vi "render hold note_pink.vi"(4 "head index":i32, 6 "progress":dbl, 7 "y-center":dbl, 10 "rail":cluster{"note type":string, "position":dbl}[](array[cluster]), 11 "new picture in":picture) -> (3 "new picture out":picture)   [LabVIEW 2023]
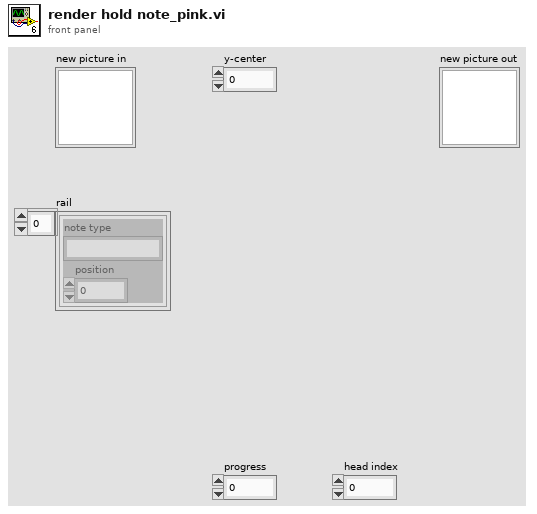
[diagram p1: front panel]
types:
  T1 = cluster{"Width":u16, "Style":enum32{"Solid", "Dash", "Dot", "DashDot", "DashDotDot"}}
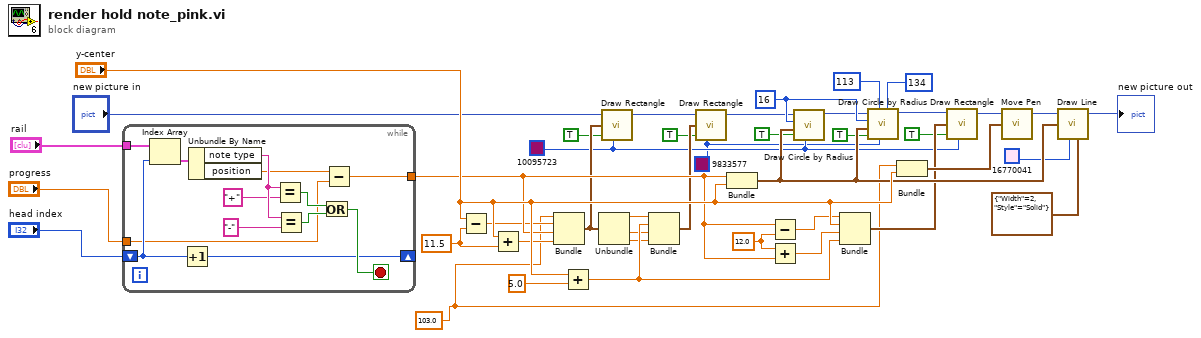
[diagram p0: block diagram]
diagram:
  w1 = 103.0 ("y")
  w4 = u32 9833577 ("color(black)")
  w5 = u32 10095723 ("color(black)")
  w31 = 12.0 ("y")
  w11 = 11.5 ("y")
  w28 = i16 16 ("radius")
  n1 = while {
    tunnel: "rail" -> [w55]
    shift-right: [w46] -> _
    shift-left: "head index" -> [w47]
    tunnel: "progress" -> [w45]
    tunnel: [w43] -> w32
    stop <- w48 stop-if-true
    n2 = Index Array(array=w55, index=w47) -> (element=w54:cluster{"note type":string, "position":dbl})
    n3 = Increment(x=w47) -> (x+1=w46:i32)
    n4 = Unbundle By Name(w54) -> ("note type"=w51:string, "position"=w44:dbl)
    n5 = Equal?(x=w51, y="+") -> (x = y?=w53:bool)
    n6 = Equal?(x=w51, y="-") -> (x = y?=w52:bool)
    n7 = Or(x=w53, y=w52) -> (x .or. y?=w48:bool)
    n8 = Subtract(x=w44, y=w45) -> (x-y=w43:dbl)
  }
  n9 = Subtract(x="y-center", y=w11) -> (x-y=w10:dbl)
  n10 = Add(x="y-center", y=w11) -> (x+y=w12:dbl)
  n11 = Bundle("y"=w1, w10, w32, w12) -> (w18:cluster{"y":dbl, dbl, dbl, dbl})  [unwired: 1 in]
  n12 = Add(x="y-center", y=5.0) -> (x+y=w35:dbl)
  n13 = Unbundle(w18) -> ("y"=w19:dbl, w20:dbl, w21:dbl)  [unwired: 1 out]
  n14 = call <vilib>:"Draw Rectangle.vi"("picture"="new picture in", "rect"=w18, "fill?(F)"=TRUE, "color(black)"=w5) -> ("new picture"=w15:picture)  [unwired: 5 in]
  n15 = Bundle("y"=w19, w35, w20, w21) -> (w23:cluster{"y":dbl, dbl, dbl, dbl})  [unwired: 1 in]
  n16 = call <vilib>:"Draw Rectangle.vi"("picture"=w15, "rect"=w23, "fill?(F)"=TRUE, "color(black)"=w4) -> ("new picture"=w16:picture)  [unwired: 5 in]
  n17 = Bundle(w32, "y-center"="y-center") -> (w40:cluster{dbl, "y-center":dbl})  [unwired: 1 in]
  n18 = Subtract(x=w32, y=w31) -> (x-y=w33:dbl)
  n19 = Add(x=w31, y=w32) -> (x+y=w34:dbl)
  n20 = call <vilib>:"Draw Circle by Radius.vi"("color(black)"=w5, "fill?(F)"=TRUE, "pixel center"=w40, "radius"=w28, "picture"=w16) -> ("new picture"=w24:picture)  [unwired: 6 in]
  n21 = Bundle(w33, "y-center"="y-center", w34, w35) -> (w36:cluster{dbl, "y-center":dbl, dbl, dbl})  [unwired: 1 in]
  n22 = call <vilib>:"Draw Circle by Radius.vi"("arc size(360)"=i16 134 ("radius"), "color(black)"=w4, "start angle(0)"=i16 113 ("radius"), "fill?(F)"=TRUE, "pixel center"=w40, "radius"=w28, "picture"=w24) -> ("new picture"=w29:picture)  [unwired: 4 in]
  n23 = Bundle("y"=w1, "y-center"="y-center") -> (w38:cluster{"y":dbl, "y-center":dbl})  [unwired: 1 in]
  n24 = call <vilib>:"Draw Rectangle.vi"("picture"=w29, "rect"=w36, "fill?(F)"=TRUE, "color(black)"=w5) -> ("new picture"=w37:picture)  [unwired: 5 in]
  n25 = call <vilib>:"Move Pen.vi"("new position"=w38, "picture"=w37) -> ("new picture"=w39:picture)  [unwired: 3 in]
  n26 = call <vilib>:"Draw Line.vi"("picture"=w39, "end point"=w40, "color(black)"=u32 16770041, "pen"=T1 {"Width"=2, "Style"=enum."Solid"}) -> ("new picture"=→"new picture out":picture)  [unwired: 5 in]
